vi "Sim Input.vi"(7 "error in (no error)":errorcluster caption="错误输入（无错误）", 9 "mode":enum16{"Get", "Set"}(ring), 10 "SW In":T1) -> (0 "error out":errorcluster caption="错误输出", 3 "SW Out":T1)   [LabVIEW 2013]
uses:
  Control/SW.ctl
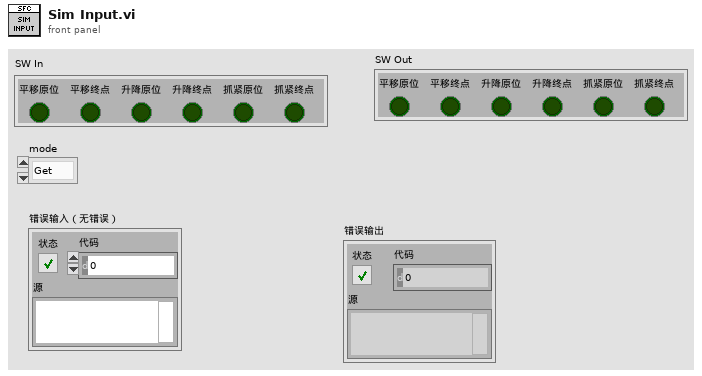
[diagram p1: front panel]
types:
  T1 = typedef "SW.ctl" = cluster{"平移原位":bool, "平移终点":bool, "升降原位":bool, "升降终点":bool, "抓紧原位":bool, "抓紧终点":bool}
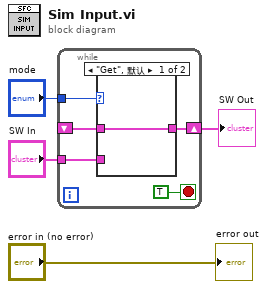
[diagram p0: block diagram]
diagram:
  n1 = while {
    tunnel: "mode" -> [w9]
    shift-right: [w5] -> w1
    shift-left: _ -> [w7]
    tunnel: "SW In" -> [w6]
    stop <- TRUE stop-if-true
    n2 = case shown="\"Get\", 默认" w9 {
      tunnel: w7 -> [w10 _]
      tunnel: w6 -> [_ w11]
      tunnel: [w10 w11] -> w5
      frame "Get", Default {
      }
      frame "Set" {
      }
    }
  }
  "SW Out" <- w1
  "error out" <- "error in (no error)"
